vi "RangeStatus.vi"(0 "VisaCluster":T2, 11 "error in (no error)":errorcluster) -> (4 "VisaCluster":T2, 8 "Answer":string, 10 "Range":T1, 15 "error out":errorcluster)   [LabVIEW 2014, in "FH 55.lvlib"]
doc: "Dieses VI gibt die Range (Messbereich) der Messwerte zurück. \n\nThis VI returns the range of the measurements."
uses:
  FH 55.lvlib
  TypeDef/VisaCluster.ctl
  TypeDef/Range.ctl
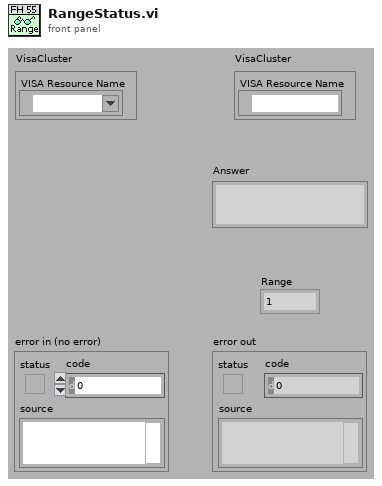
[diagram p1: front panel]
types:
  T1 = typedef "FH 55.lvlib/Range.ctl" = enum16{"1", "2", "3", "4", "5", "6", "7"}
  T2 = typedef "FH 55.lvlib/VisaCluster.ctl" = cluster{"VISA Resource Name":refnum<visa-resource-name>}
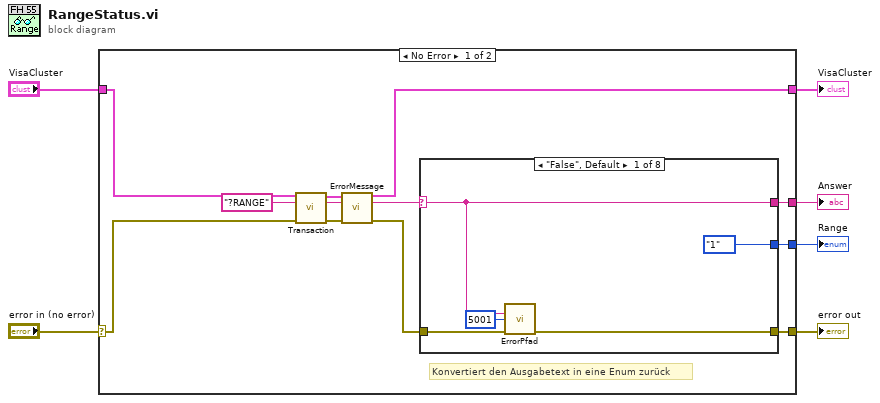
[diagram p0: block diagram]
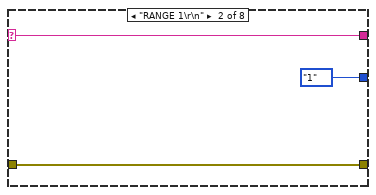
[diagram p2: hidden frame]
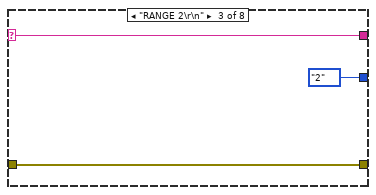
[diagram p3: hidden frame]
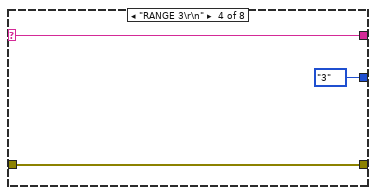
[diagram p4: hidden frame]
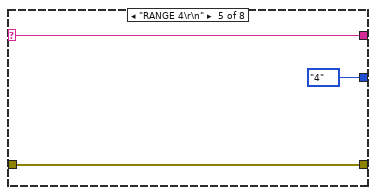
[diagram p5: hidden frame]
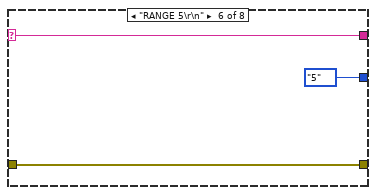
[diagram p6: hidden frame]
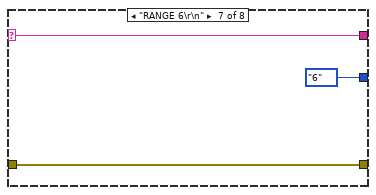
[diagram p7: hidden frame]
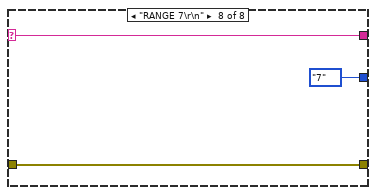
[diagram p8: hidden frame]
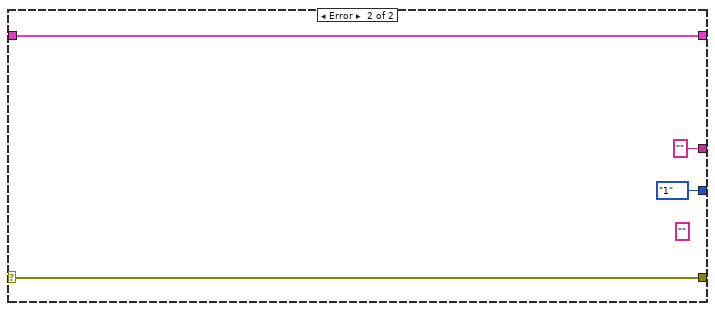
[diagram p9: hidden frame]
diagram:
  n1 = case shown="No Error" "error in (no error)" {
    selector: "error in (no error)" -> [w7 w47]
    tunnel: "VisaCluster" -> [w8 w48]
    tunnel: [w18 w48] -> w2
    tunnel: [w13 w47] -> w4
    tunnel: [w12 ""] -> w3
    tunnel: [w9 Range."1" ("Range")] -> w1
    frame No Error {
      # "Konvertiert den Ausgabetext in eine Enum zurück"
      n2 = call "Transaction.vi"("VisaCluster"=w8, "Command"="?RANGE", "error in (no error)"=w7) -> ("VisaCluster"=w16:T2, "Answer"=w11:string, "error out"=w17:errorcluster)  [unwired: 9 in, 1 out]
      n3 = call "ErrorMessage.vi"("VisaCluster"=w16, "Message In"=w11, "error in (no error)"=w17) -> ("VisaCluster"=w18:T2, "Message Out"=w10:string, "error out"=w14:errorcluster)  [unwired: 10 in]
      n4 = case shown="\"False\", Default" w10 {
        selector: w10 -> [w21 w26 w29 w32 w35 w38 w41 w44]
        tunnel: w14 -> [w23 w25 w28 w31 w34 w37 w40 w43]
        tunnel: [w22 w25 w28 w31 w34 w37 w40 w43] -> w13
        tunnel: [w21 w26 w29 w32 w35 w38 w41 w44] -> w12
        tunnel: [Range."1" ("Range") Range."1" ("Range") Range."2" ("Range") Range."3" ("Range") Range."4" ("Range") Range."5" ("Range") Range."6" ("Range") Range."7" ("Range")] -> w9
        frame "False", Default {
          n5 = call "ErrorPfad.vi"("Message In"=w21, "Numeric"=5001, "error in (no error)"=w23) -> ("error out"=w22:errorcluster)  [unwired: 11 in, 1 out]
        }
        frame "RANGE 1\r\n" {
        }
        frame "RANGE 2\r\n" {
        }
        frame "RANGE 3\r\n" {
        }
        frame "RANGE 4\r\n" {
        }
        frame "RANGE 5\r\n" {
        }
        frame "RANGE 6\r\n" {
        }
        frame "RANGE 7\r\n" {
        }
      }
    }
    frame Error {
      (unwired) ""
    }
  }
  "error out" <- w4
  "Answer" <- w3
  "VisaCluster" <- w2
  "Range" <- w1
